vi "Choose Controller.vi"(8 "error in (no error)":errorcluster, 11 "ctlr queue":refnum<queue>) -> (0 "error out":errorcluster)   [LabVIEW 2020]
uses:
  Controller Loop/Message and Data.ctl
  Inflation Test/Parameter Class/IA Test Parameters.lvclass
  Controller.lvclass
  Hardware/Sensors/Cameras/Camera.lvclass
  Hardware/Sensors/Force Sensors/Force Sensor.lvclass
  Hardware/Actuators/Servos/Servo.lvclass
  Hardware/Actuators/Switches/Switch.lvclass
  File Interfacing/Filename Structure.ctl
  Simulated Controller/Simulated Controller.lvclass
  C:/Users/Haslach/Documents/Inflation-Apparatus/src/Controllers/Controller.lvclass
  PID/PID Controller.lvclass
  PID/PID Controller.lvclass/PID Controller.ctl
  Controller.lvclass/Controller.ctl
  Write PW Limits.vi
  Open-loop Controller/Open-loop Controller.lvclass
  C:/Users/Haslach/Documents/Inflation-Apparatus/src/Controllers/Simulated Controller/Simulated Controller.lvclass
  C:/Users/Haslach/Documents/Inflation-Apparatus/src/Controllers/PID/PID Controller.lvclass
  C:/Users/Haslach/Documents/Inflation-Apparatus/src/Controllers/Open-loop Controller/Open-loop Controller.lvclass
panel:
  in  "discard":bool
  in  "continue":bool
  in  "controller tab":T1(tab)=enum."PID Controller"
  in  "PID gains":T2={"proportional gain (Kc)"=1.0, "integral time (Ti, min)"=0.01, "derivative time (Td, min)"=0.0} caption="PID GAINS" {"derivative time (Td, min)" format="%.3f"; "integral time (Ti, min)" format="%.3f"; "proportional gain (Kc)" format="%.3f"}
  # "CONTROLLER SELECTION"
  # "NO CONTROLLER WILL BE USED, GENERATED PULSES WILL BE RANDOM"
  # "NO CONTROLLER WILL BE USED, \nPULSES WILL BE EQUAL TO TEST PARAMTERS"
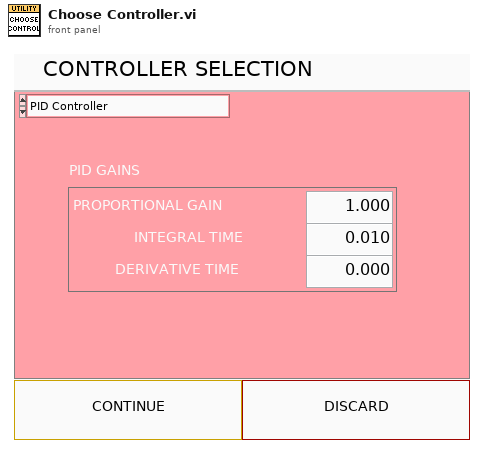
[diagram p1: front panel]
types:
  T1 = enum32{"Simulated Controller", "PID Controller", "Open-loop Controller"}
  T2 = cluster{"proportional gain (Kc)":dbl, "integral time (Ti, min)":dbl, "derivative time (Td, min)":dbl}
  T3 = typedef "Message and Data.ctl" = cluster{"msg":string, "ia test param":refnum<class "IA Test Parameters.lvclass">, "controller type":refnum<class "Controller.lvclass">, "folder path":path, "file name":string, "file comments":string, "cam":refnum<class "Camera.lvclass">, "fs":refnum<class "Force Sensor.lvclass">, "servo":refnum<class "Servo.lvclass">, "switch":refnum<class "Switch.lvclass">, "filename struct":T4, "mm/pixel":dbl, "rectangle":T5}
  T4 = typedef "Filename Structure.ctl" = enum16{"<nameYYYYMMDDi>", "<name>"}
  T5 = typedef "IMAQ Rectangle" = cluster{"Left":i32, "Top":i32, "Right":i32, "Bottom":i32, "Rotation":dbl}
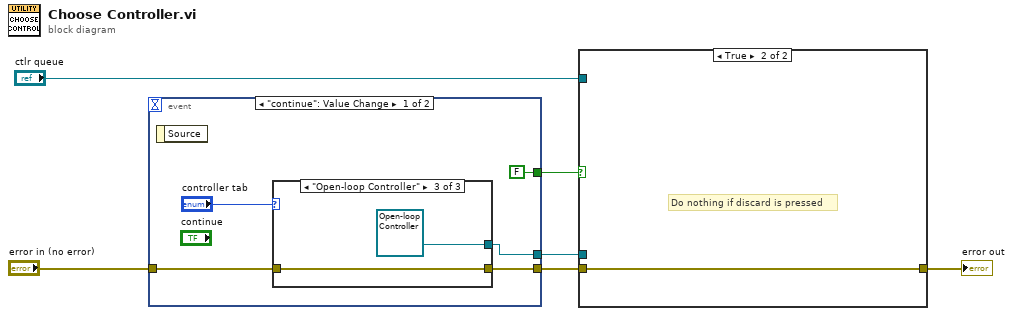
[diagram p0: block diagram]
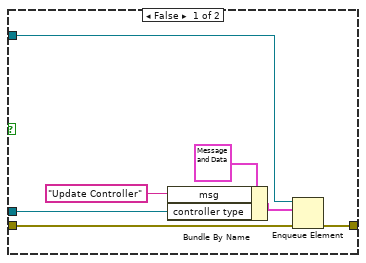
[diagram p2: hidden frame]
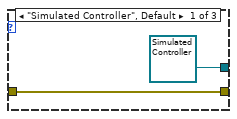
[diagram p3: hidden frame]
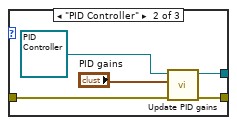
[diagram p4: hidden frame]
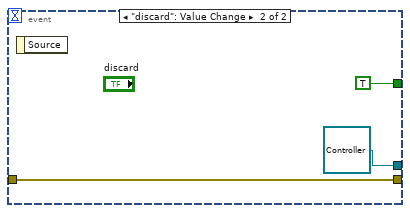
[diagram p5: hidden frame]
diagram:
  n1 = event shown="[0] \"continue\": Value Change" {
    selector: _ -> [_ _]
    dyn-events: _ -> [_ _]
    timeout: _ -> [_ _]
    tunnel: "error in (no error)" -> [w11 w23]
    tunnel: [w10 w23] -> w3
    tunnel: [w9 refnum<class "Controller.lvclass"> refnum ("PID Controller out")] -> w2
    tunnel: [FALSE TRUE] -> w1
    event "continue": Value Change {
      n2 = event-data() -> ()  [unwired: 1 in, 1 out]
      n3 = case shown="\"Open-loop Controller\"" "controller tab" {
        tunnel: [refnum<class "Simulated Controller.lvclass"> refnum ("Simulated Controller.lvclass") w17 refnum<class "Open-loop Controller.lvclass"> refnum ("Open-loop Controller.lvclass")] -> w9
        tunnel: w11 -> [w12 w16 w20]
        tunnel: [w12 w15 w20] -> w10
        frame "Simulated Controller", Default {
        }
        frame "PID Controller" {
          n4 = call "Update PID gains.vi"("error in (no error)"=w16, "PID gains"="PID gains", "PID Controller in"=refnum<class "PID Controller.lvclass"> refnum ("PID Controller.lvclass")) -> ("error out"=w15:errorcluster, "PID Controller out"=w17:refnum<class "PID Controller.lvclass">)  [unwired: 7 in]
        }
        frame "Open-loop Controller" {
        }
      }
    }
    event "discard": Value Change {
      n5 = event-data() -> ()  [unwired: 1 in, 1 out]
    }
  }
  n6 = case shown="True" w1 {
    tunnel: [w29 w31] -> w6
    tunnel: "ctlr queue" -> [w28 _]
    tunnel: w3 -> [w25 w31]
    tunnel: w2 -> [w24 _]
    frame False {
      n7 = Bundle By Name(cluster=T3 {"msg"="", "ia test param"=refnum, "controller type"=refnum, "folder path"=path "", "file name"="", "file comments"="", "cam"=refnum, "fs"=refnum, "servo"=refnum, "switch"=refnum, "filename struct"=enum."<nameYYYYMMDDi>", "mm/pixel"=0.0, "rectangle"={"Left"=0, "Top"=0, "Right"=0, "Bottom"=0, "Rotation"=0.0}} ("element"), "msg"="Update Controller", "controller type"=w24) -> (w27:T3)
      n8 = Enqueue Element(queue=w28, element=w27, error in (no error)=w25) -> (error out=w29:errorcluster)  [unwired: 1 in, 2 out]
    }
    frame True {
      # "Do nothing if discard is pressed"
    }
  }
  "error out" <- w6
